vi "array.vi"() -> ()   [LabVIEW 2020]
panel:
  out "initialized array":dbl[][](array[numeric])
  out "appended array 2":string[][](array[string])
  out "appended array":string[](array[string])
  out "reversed array":string[](array[string])
  out "array w/ subset deleted 2":i32[][](array[numeric])
  out "deleted portion":string[](array[string])
  out "array w/ subset deleted":string[](array[string])
  out "output array 2":string[](array[string])
  out "size(s) 2":i32
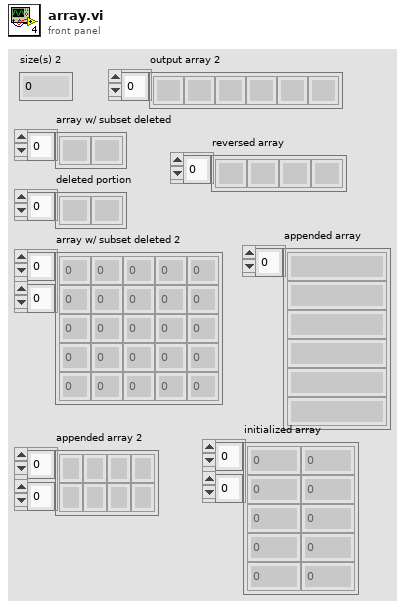
[diagram p1: front panel]
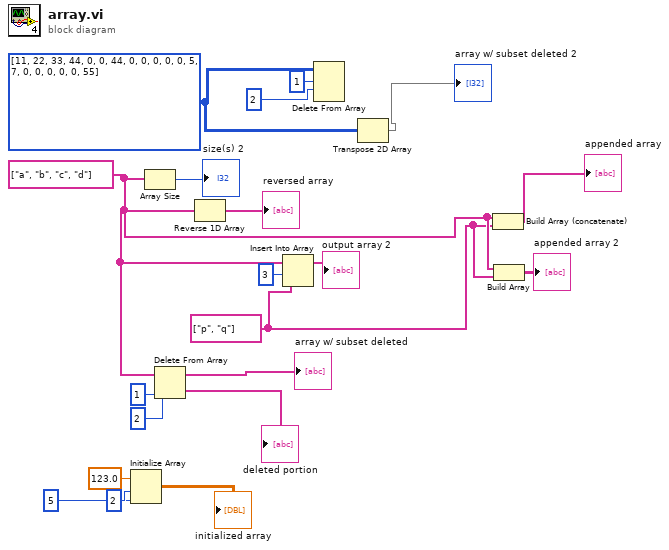
[diagram p0: block diagram]
diagram:
  w6 = string[] ["p", "q"]
  w10 = i32[][] [[11, 22, 33, 44, 0], [0, 44, 0, 0, 0], [0, 0, 5, 7, 0], [0, 0, 0, 0, 55]] ("Array")
  w7 = string[] ["a", "b", "c", "d"]
  n1 = Initialize Array(123.0 ("element"), 5 ("dimension size"), 2 ("dimension size")) -> (→"initialized array":dbl[][])
  n2 = Array Size(array=w7) -> (size(s)=→"size(s) 2":i32)
  n3 = Delete From Array(array=w7, length=2, index=1) -> (deleted portion=→"deleted portion":string[], array with subset deleted=→"array w/ subset deleted":string[])
  n4 = Reverse 1D Array(array=w7) -> (reversed array=→"reversed array":string[])
  n5 = Insert Into Array(array=w7, index=3, new element=w6) -> (→"output array 2":string[])
  n6 = Delete From Array(array=w10, length=1, index (row)=2 ("disabled index (col)")) -> ()  [unwired: 1 in, 2 out]
  n7 = Transpose 2D Array(2D array=w10) -> (transposed array=→"array w/ subset deleted 2":i32[][])
  n8 = Build Array (concatenate)(w7, w6) -> (→"appended array":string[])
  n9 = Build Array(w7, w6) -> (→"appended array 2":string[][])
